vi "Get_Dbl_Coordinates_From_Map_Cell (SubVI).vi"(9 "Y_map":i32, 10 "X_map":i32) -> (1 "Y":dbl, 2 "X":dbl)   [LabVIEW 2017]
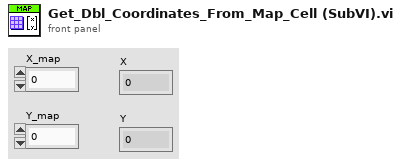
[diagram p1: front panel]
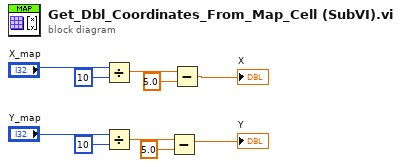
[diagram p0: block diagram]
diagram:
  n1 = Divide(x="X_map", y=10) -> (x/y=w6:dbl)
  n2 = Divide(x="Y_map", y=10) -> (x/y=w4:dbl)
  n3 = Subtract(x=w4, y=5.0) -> (x-y=→"Y":dbl)
  n4 = Subtract(x=w6, y=5.0) -> (x-y=→"X":dbl)
